vi "SwerveKinematics_ToSwerveModuleStatesZeroCenter.vi"(10 "ChassisSpeeds":T6 {"vOmega" format="%10.3f"; "vY" format="%10.3f"; "vX" format="%10.3f"}, 11 "in SWERVE_DRIVE_KINEMATICS":T3 {"PrevCoR"."Y" format="%14.3f"; "PrevCoR"."X" format="%14.3f"; "Modules"."Y" format="%14.3f"; "Modules"."X" format="%14.3f"}) -> (1 "ModuleStates":T1[](array[typedef]) {"Angle"."SIN" format="%13.4f"; "Angle"."COS" format="%13.4f"; "Angle"."VALUE" format="%13.4f"}, 3 "out SWERVE_DRIVE_KINEMATICS":T3 {"PrevCoR"."Y" format="%14.3f"; "PrevCoR"."X" format="%14.3f"; "Modules"."Y" format="%14.3f"; "Modules"."X" format="%14.3f"})   [LabVIEW 2019, in "Trajectory_Library.lvlib"]
doc: "Performs inverse kinematics to return the module states from a desired chassis velocity. This method is often used to convert joystick values into module speeds and angles.\n \nThis uses the robot center as the center of rotation. During normal operations, the center of rotation is usually the same as the physical center of the robot; therefore, the argument is defaulted to that use case. However, if you wish to change the center of rotation for evasive manuevers, vision alignment, or for any other use case, you can do so.\n \nParameters:\n - chassisSpeeds -- The desired chassis speed.\n\nReturns:\n - ModuleStates - An array of data structures containing the module states. Use caution because these module states are not normalized. Sometimes, a user input may cause one of the module speeds to go above the attainable max velocity. Use the {@link #normalizeWheelSpeeds(SwerveModuleState[], double) normalizeWheelSpeeds} function to rectify this issue."
uses:
  Trajectory_Library.lvlib
  TypeDef/SWERVE_DRIVE_KINEMATICS.ctl
  <vilib>/Analysis/Matrix/Datatypes/RealMatrix.ctl
  TypeDef/TRANSLATION2D.ctl
  TypeDef/CHASSIS_SPEEDS.ctl
  TypeDef/SWERVE_DRIVE_MODULE_STATE.ctl
  TypeDef/ROTATION2D.ctl
  <vilib>/Analysis/Matrix/NI_Matrix.lvlib
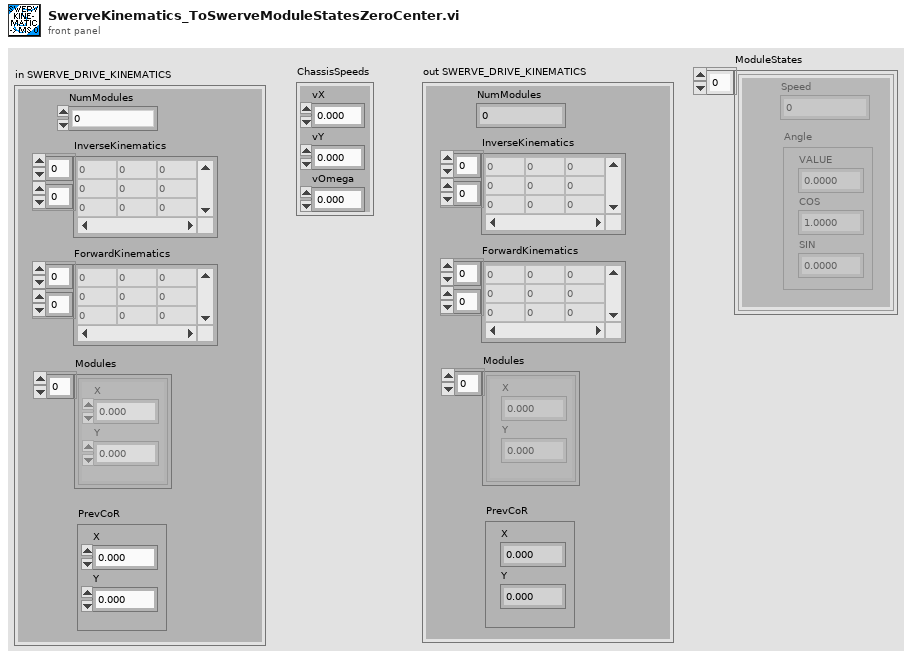
[diagram p1: front panel]
types:
  T1 = typedef "Trajectory_Library.lvlib/SWERVE_DRIVE_MODULE_STATE.ctl" = cluster{"Speed":dbl, "Angle":T2}
  T2 = typedef "Trajectory_Library.lvlib/ROTATION2D.ctl" = cluster{"VALUE":dbl, "COS":dbl, "SIN":dbl}
  T3 = typedef "Trajectory_Library.lvlib/SWERVE_DRIVE_KINEMATICS.ctl" = cluster{"NumModules":i32, "InverseKinematics":T4, "ForwardKinematics":T4, "Modules":T5[], "PrevCoR":T5}
  T4 = typedef "NI_Matrix.lvlib/RealMatrix.ctl" = dbl[][]
  T5 = typedef "Trajectory_Library.lvlib/TRANSLATION2D.ctl" = cluster{"X":dbl, "Y":dbl}
  T6 = typedef "Trajectory_Library.lvlib/CHASSIS_SPEEDS.ctl" = cluster{"vX":dbl, "vY":dbl, "vOmega":dbl}
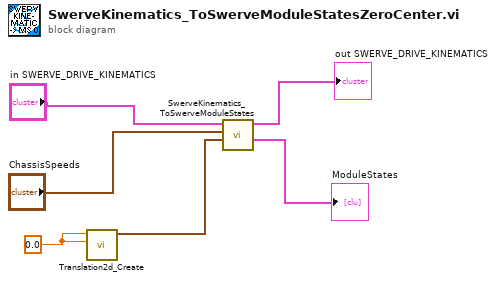
[diagram p0: block diagram]
diagram:
  w4 = 0.0 ("X")
  n1 = call "Translation2d_Create.vi"("Y"=w4, "X"=w4) -> ("TRANSLATION"=w3:T5)  [unwired: 9 in]
  n2 = call "SwerveKinematics_ToSwerveModuleStates.vi"("CenterOfRotation"=w3, "ChassisSpeeds"="ChassisSpeeds", "in SWERVE_DRIVE_KINEMATICS"="in SWERVE_DRIVE_KINEMATICS") -> ("ModuleStates"=→"ModuleStates":T1[], "out SWERVE_DRIVE_KINEMATICS"=→"out SWERVE_DRIVE_KINEMATICS":T3)  [unwired: 7 in]
